vi "trigger_test_host.vi"() -> ()   [LabVIEW 2014]
uses:
  <vilib>/userdefined/High Color/nirio_resource_hc.ctl
  <vilib>/FPGAPlugInAG/PXIe-7962R/niLvFpga_Open_PXIe-7962R.vi
  <vilib>/rvi/interface/common/dynamic/niFpgaDynamicAddResources.vi
  <instrlib>/_niInstr/Streaming/v1/Host/Public/Start Finite Stream.vi
  <instrlib>/niSync/niSync.llb/niSync Initialize (IVI).vi
  <vilib>/Utility/error.llb/Error Cluster From Error Code.vi
  <vilib>/rvi/errors/niLvFpgaAdjustHostInterfaceError.vi
  <vilib>/FPGAPlugInAG/Dynamic/niLvFpga_Close_Dynamic.vi
  <vilib>/rvi/interface/nirviOpenFPGA/nirviOpenFPGA.xnode
  FPGA Bitfiles/MochiFPGAControl_FPGATarget_fpgatriggertest_l4hEgdtRZUI.lvbitx
  <vilib>/rvi/interface/nirviReadWriteControl/nirviReadWriteControl.xnode
  <vilib>/rvi/interface/nirviCloseFPGA/nirviCloseFPGA.xnode
  <instrlib>/_niInstr/Streaming/v1/Host/niInstr Streaming v1 Host.lvlib
  NiFpgaLv.dll
  <vilib>/rvi/interface/Simulation/niFpgaSimulationCallBeginRW.vi
panel:
  out "count out":u64
  out "trigger active?":bool
  out "request data":bool
  out "send data":bool
  in  "resource name":T1 caption="RIO Device"
  in  "destination terminal":string(combo)="PXI_Trig0"
  in  "Trigger?":bool
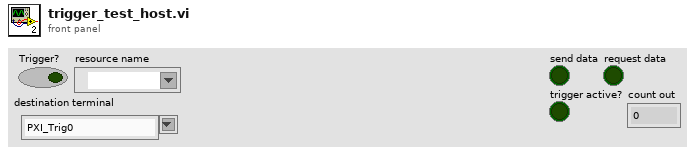
[diagram p1: front panel]
types:
  T1 = typedef "nirio_resource_hc.ctl" = tag
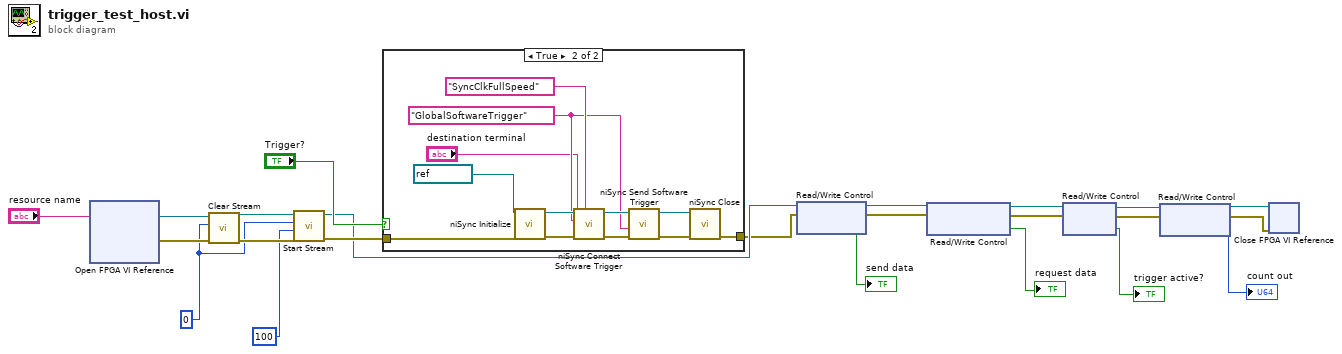
[diagram p0: block diagram]
diagram:
  w1 = 0 ("stream index")
  n1 = xnode "Open FPGA VI Reference"("resource name"="resource name") -> ("FPGA VI Reference Out"=w23:refnum<k20>, "error out"=w22:errorcluster)  [unwired: 1 in]
  n2 = call <instrlib>:"Clear Stream.vi"("error in (no error)"=w22, "stream index"=w1, "refnum in"=w23) -> ("error out"=w20:errorcluster, "refnum out"=w21:refnum<k20>)  [unwired: 7 in]
  n3 = call-poly <instrlib>:"Start Stream.vi"("error in (no error)"=w20, "num samples"=u64 100, "stream index"=w1, "refnum in"=w21) -> ("error out"=w17:errorcluster, "refnum out"=w15:refnum<k20>)  [unwired: 6 in]
  n4 = case shown="True" "Trigger?" {
    tunnel: w17 -> [w24 w27]
    tunnel: [w24 w26] -> w10
    frame False {
    }
    frame True {
      w28 = "GlobalSoftwareTrigger" ("source terminal")
      n5 = call-poly <instrlib>:"niSync Initialize.vi"("error in (no error)"=w27, "resource name"=refnum<k15> "Sync0") -> ("error out"=w36:errorcluster, "instrument handle out"=w35:refnum<k15>)  [unwired: 8 in]
      n6 = call <instrlib>:"niSync Connect Software Trigger.vi"("synchronization clock"="SyncClkFullSpeed", "error in (no error)"=w36, "destination terminal"="destination terminal", "source terminal"=w28, "instrument handle"=w35) -> ("error out"=w34:errorcluster, "instrument handle out"=w33:refnum<k15>)  [unwired: 5 in]
      n7 = call <instrlib>:"niSync Send Software Trigger.vi"("error in (no error)"=w34, "source terminal"=w28, "instrument handle"=w33) -> ("error out"=w31:errorcluster, "instrument handle out"=w32:refnum<k15>)  [unwired: 7 in]
      n8 = call <instrlib>:"niSync Close.vi"("error in (no error)"=w31, "instrument handle"=w32) -> ("error out"=w26:errorcluster)  [unwired: 9 in]
    }
  }
  n9 = xnode "Read/Write Control"("FPGA VI Reference In"=w15, "error in"=w10) -> ("FPGA VI Reference Out"=w14:refnum<k20>, "error out"=w11:errorcluster, "send data"=→"send data":bool)
  n10 = xnode "Read/Write Control"("FPGA VI Reference In"=w14, "error in"=w11) -> ("FPGA VI Reference Out"=w9:refnum<k20>, "error out"=w8:errorcluster, "request data"=→"request data":bool)
  n11 = xnode "Read/Write Control"("FPGA VI Reference In"=w9, "error in"=w8) -> ("FPGA VI Reference Out"=w6:refnum<k20>, "error out"=w5:errorcluster, "out"=→"trigger active?":bool)
  n12 = xnode "Read/Write Control"("FPGA VI Reference In"=w6, "error in"=w5) -> ("FPGA VI Reference Out"=w3:refnum<k20>, "error out"=w2:errorcluster, "count out"=→"count out":u64)
  n13 = xnode "Close FPGA VI Reference"("FPGA VI Reference In"=w3, "error in"=w2) -> ()  [unwired: 1 out]
